vi "SIMCOMCommunicationTool_CF_vb.vi"(0 "VISA资源名称":refnum<visa-resource-name>="COM26", 1 "MSComm":refnum<k7>, 2 "MEID":string, 5 "通信协议名称":string, 9 "DelayTime":u32=100, 11 "error in":errorcluster, 12 "Debug":bool=TRUE, 14 "Slot":T1) -> (3 "CMD":string="发送 重启:AT+CRESET\r反馈:\r\nOK\r\n\r\n", 4 "字符串数值":bool=TRUE, 6 "反馈结果":bool=TRUE, 10 "ReturnData":string, 15 "error out":errorcluster)   [LabVIEW 2013]
doc: "本范例根据用户指示，对串口执行读写操作。范例运行时可按下“写入”或“读取”按钮，以及修改“读数”。\n\n设置的串口参数必须匹配连接仪器或设备的参数。本范例中，“读数”参数可指定串口读取的字节数。如端口字节超过指定的字节数，超出部分将不会被读取。如端口字节数少于指定的字节数，将返回超时错误。\n\n本范例可扩展流控制选项以包括XON和XOFF，从而允许用户选择控制字符。同时，用户可启用或禁用中止符。部分设备需要通过终止符确定命令字符串的结束位置。部分设备将发送终止符以说明待读取数据的末端。本范例演示了缓冲区中检测到终止符时，结束“读取”操作或添加终止符至“写入”数据末端的方法。"
uses:
  SystemCode/SysControl/Slot.ctl
  <vilib>/Utility/NIReport.llb/NI_report.lvclass
  SourceCode/GlobalValue.vi
  <vilib>/Utility/error.llb/Error Cluster From Error Code.vi
  <vilib>/addons/_office/excel.llb/Excel Get Data ([str]).vi
  <vilib>/ErrorRing/Error Ring.xnode
  <vilib>/addons/_office/NI_ReportGenerationToolkit.lvlib
  <vilib>/Utility/NIReport.llb/Excel/NI_Excel.lvclass
panel:
  out "Data":string[][](array[string])=[["8986031490021881534", "460036161669975", "2A645416CB435F94", "8006A127", "460036161669975@mycdma.cn", "DB60264368A1D188", "18101891253", "A1000021A59070"], ["8986031490021881535", "460036161669976", "32FA5764D69C76BE", "80FAE4E6", "460036161669976@mycdma.cn", "B3AA1B3D2F0D5593", "18964872399", "A1000021A58D61"], ["", "", "", "", "", "", "", ""], ["", "", "", "", "", "", "", ""], ["", "", "", "", "", "", "", ""], ["", "", "", "", "", "", "", ""], ["", "", "", "", "", "", "", ""], ["", "", "", "", "", "", "", ""], ["", "", "", "", "", "", "", ""], ["", "", "", "", "", "", "", ""], ["", "各位，模块烧号主要是写五码，包括IMSI、AKEY、MEID（ESN）、AN(EVDO USER)、AAA(EVDO PWD)。", "", "", "", "", "", ""], ["", "其中ESN和MEID在模块出厂时已经写入，两者均可通过AT指令读取，但ESN不可更改。", "", "", "", "", "", ""], ["", "经询问及实际测试，上海电信绑定ESN号而广东电信未绑定，意味着上海电信五码烧录到其它模块是不可用的，但广东电信则无此限制。", "", "", "", "", "", ""], ["", "", "", "", "", "", "", ""], ["", "", "", "", "", "", "", ""], ["", "目前已确定跟上海电信合作，后续模块及卡号使用过程中，如遇到模块损坏，则意味着该卡必须销号（除非向电信申请绑定新的ESN），否则烧录到其它模块中是没用的。", "", "", "", "", "", ""]]
  in  "命令列表":u16(ring)=18 items=["查询RTRECF", "设置RTRECF", "查询MEID", "设置MEID", "查询ESN", "设置ESN", "查询AKEY", "设置AKEY", "查询IMSI1", "设置IMSI1", "查询IMSI2", "设置IMSI2", "查询IMSI3", "设置IMSI3", "设置EVDO账号", "设置EVDO密码", "打开音频LOOPBACK", "关闭音频LOOPBACK", "重启", "打开网络", "查询网络状态", "连网测试", "查询CIP", "切换声音通道", "测试登录", "拨号", "挂断", "查询IP", "AT+CSOCKAUTHNV", "AT+CSOCKAUTH", "查询2G信号", "查询3G信号", "H330测试通讯", "H330打开音频回环", "H330关闭音频回环", "H330拨号"]
  out "ConfigPath":string="D:\\导航\\T-BOX\\新建文件夹\\config\\通信协议.xls"
  out "DataType":string="AT+CRESET"
  out "命令":string="AT+CRESET\r"
  out "响应":string="\r\nOK\r\n"
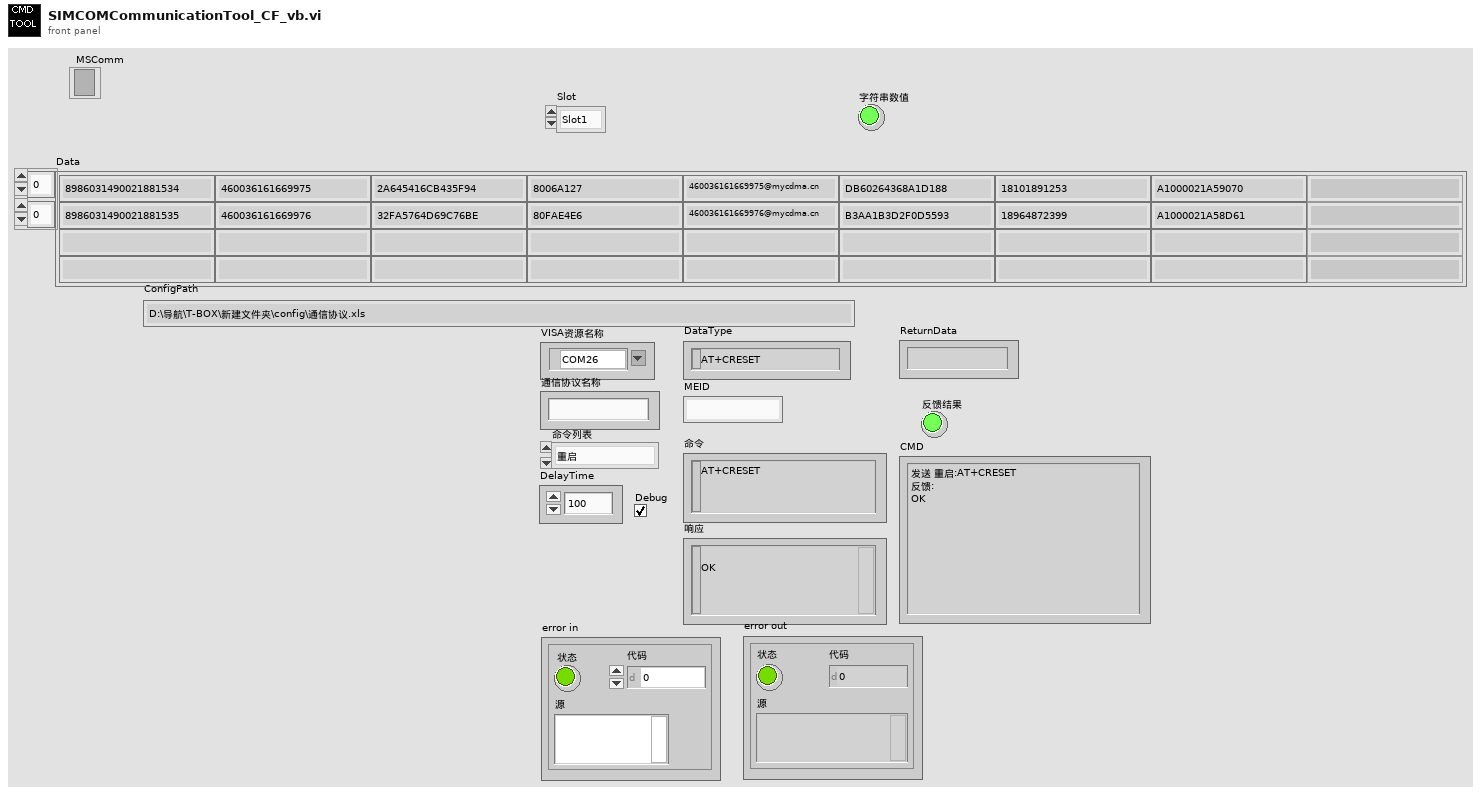
[diagram p1: front panel]
types:
  T1 = typedef "Slot.ctl" = enum16{"Slot1", "Slot2", "Slot3", "Slot4"}
  T2 = enum32{"invalid app kind", "Development System", "Run Time System", "Student Edition", "Embedded LabVIEW", "Evaluation", "Custom"}
  T3 = enum16{"maximized", "minimized", "normal", "no change"}
  T4 = enum16{"Standard Report", "HTML", "Word", "Excel"}
  T5 = cluster{"IMSI":string, "AKEY":string, "ESN":string, "EVDO账号":string, "EVDO密码":string, "设备号":string}
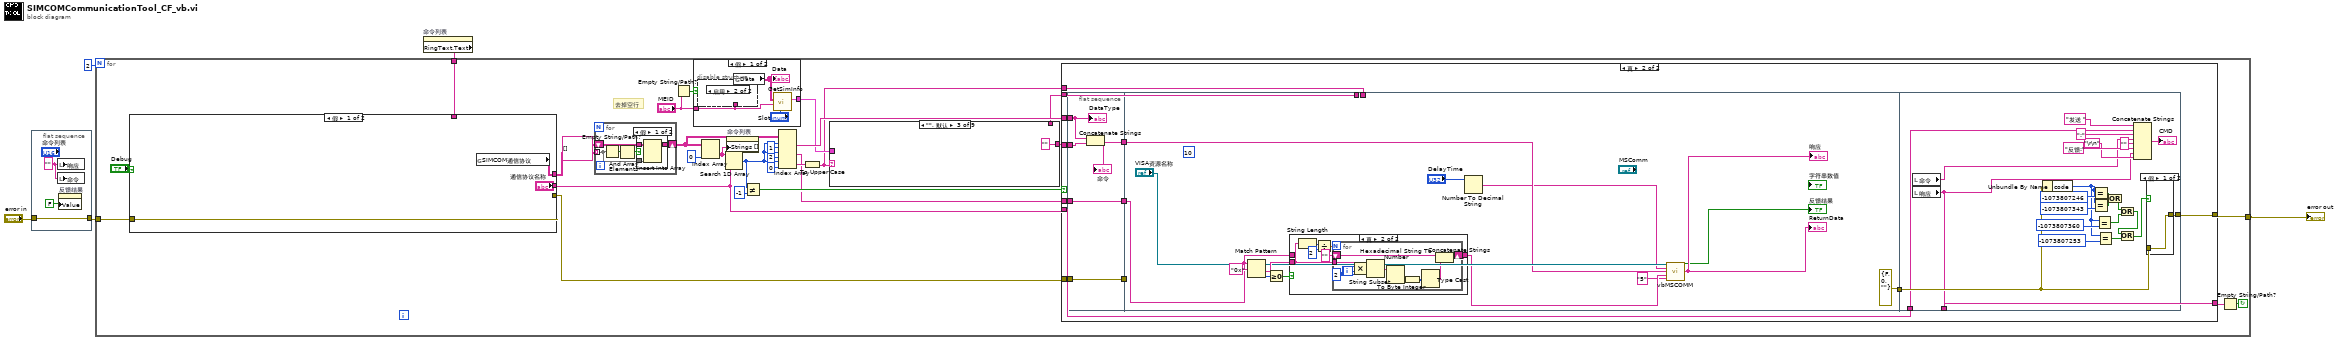
[diagram p0: block diagram]
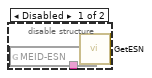
[diagram p2: hidden frame]
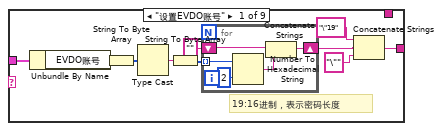
[diagram p5: hidden frame]
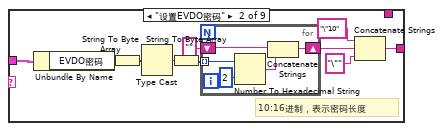
[diagram p6: hidden frame]
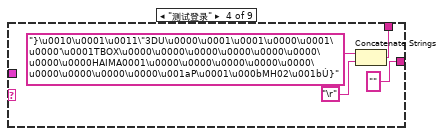
[diagram p7: hidden frame]
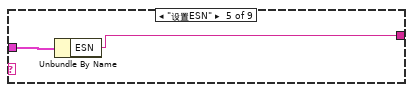
[diagram p8: hidden frame]
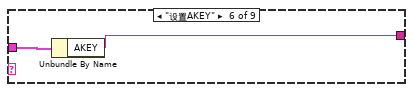
[diagram p9: hidden frame]
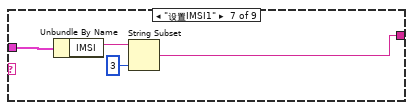
[diagram p10: hidden frame]
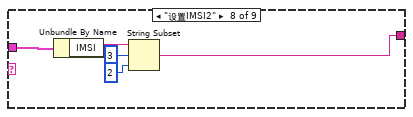
[diagram p11: hidden frame]
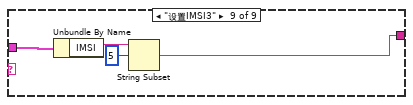
[diagram p12: hidden frame]
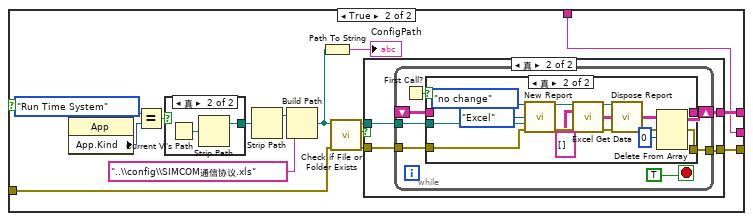
[diagram p13: hidden frame]
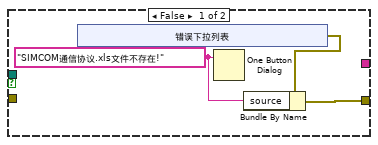
[diagram p14: hidden frame]
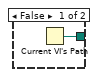
[diagram p16: hidden frame]
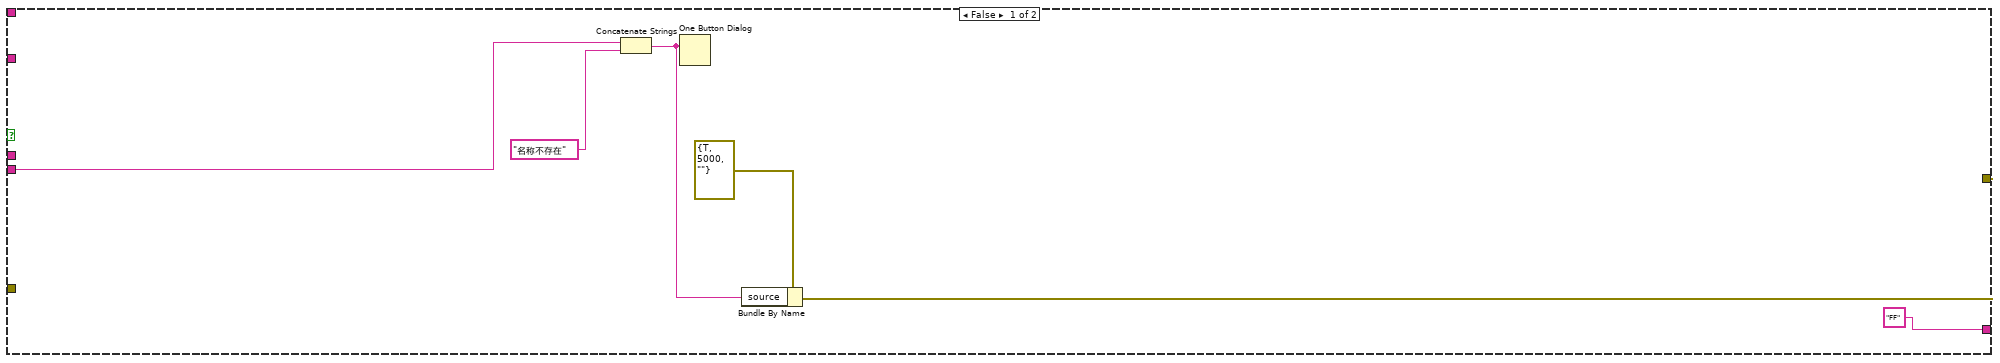
[diagram p17: hidden frame]
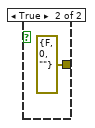
[diagram p19: hidden frame]
diagram:
  n1 = flat-sequence {
    tunnel: "error in" -> [w7]
    tunnel: [w7] -> w2
    frame #0 {
      w8 = "" ("响应")
      n2 = local write "响应"(w8) -> ()
      n3 = local write "命令"(w8) -> ()
      n4 = property on="反馈结果" class="Bool (严格)"("Value"=FALSE ("反馈结果")) -> ()  [unwired: 2 in, 2 out]
    }
  }
  n5 = property on="命令列表" class="Ring (严格)"() -> ("RingText.Text"=w1:string)  [unwired: 2 in, 2 out]
  n6 = for {
    N: 2 -> [_]
    tunnel: w2 -> [w24]
    tunnel: [w36] -> w5
    tunnel: w1 -> [w17]
    stop <- w22 continue-if-true
    # "去掉空行"
    n7 = case shown="假" "Debug" {
      tunnel: [w105 w110] -> w35
      tunnel: w24 -> [w105 w109]
      tunnel: ["通信协议名称" w107] -> w28
      tunnel: [w104 w108] -> w19
      tunnel: w17 -> [_ w107]
      frame False {
        n8 = global read "GlobalValue.vi" "SIMCOM通信协议"() -> (w104:string[][])
      }
      frame True {
        n9 = property class="App"() -> ("App.Kind"=w119:T2)  [unwired: 2 in, 2 out]
        n10 = Equal?(x=T2."Run Time System" ("y"), y=w119) -> (x = y?=w121:bool)
        n11 = case shown="真" w121 {
          tunnel: [w155 w157] -> w120
          frame False {
            n12 = Current VI's Path() -> (path=w155:path)
          }
          frame True {
            n13 = Current VI's Path() -> (path=w156:path)
            n14 = Strip Path(path=w156) -> (stripped path=w157:path)  [unwired: 1 out]
          }
        }
        n15 = Strip Path(path=w120) -> (stripped path=w114:path)  [unwired: 1 out]
        n16 = Build Path(base path=w114, name or relative path="..\\config\\SIMCOM通信协议.xls" ("连接的字符串")) -> (appended path=w116:path)
        n17 = Path To String(path=w116) -> (string=→"ConfigPath":string)
        n18 = call <vilib>:"Check if File or Folder Exists.vi"("error in (no error)"=w109, "path"=w116) -> ("error out"=w111:errorcluster, "file or folder exists?"=w113:bool, "dup path"=w112:path)  [unwired: 7 out]
        n19 = case shown="真" w113 {
          tunnel: w112 -> [_ w132]
          tunnel: w111 -> [_ w131]
          tunnel: [w123 w130] -> w110
          tunnel: [_ w129] -> w108
          frame False {
            w124 = "SIMCOM通信协议.xls文件不存在!" ("消息")
            n20 = xnode "错误下拉列表"() -> ("错误输出"=w122:errorcluster)
            n21 = One Button Dialog(message=w124) -> ()  [unwired: 1 in, 1 out]
            n22 = Bundle By Name(cluster=w122, "source"=w124) -> (w123:errorcluster)
          }
          frame True {
            n23 = while {
              tunnel: w132 -> [w138]
              tunnel: [w137] -> w130
              tunnel: w131 -> [w136]
              shift-right: [w139] -> w129
              shift-left: _ -> [w134]
              stop <- TRUE stop-if-true
              n24 = First Call?() -> (First Call?: T/F=w133:bool)
              n25 = case shown="真" w133 {
                tunnel: [w141 w145] -> w139
                tunnel: w138 -> [_ w144]
                tunnel: [w140 w143] -> w137
                tunnel: w136 -> [w140 w142]
                tunnel: w134 -> [w141 _]
                frame False {
                }
                frame True {
                  n26 = call <vilib>:"New Report.vi"("window state (normal)"=T3."no change", "report type"=T4."Excel", "template (empty)"=w144, "error in (no error)"=w142) -> ("report out"=w150:refnum<class "NI_report.lvclass">, "error out"=w151:errorcluster)  [unwired: 2 in, 8 out]
                  n27 = call-poly <vilib>:"Excel Get Data.vi"("report in"=w150, "data type"=string[][] [], "error in (no error)"=w151) -> ("report out"=w147:refnum<class "NI_report.lvclass">, "data"=w152:string[][], "error out"=w146:errorcluster)  [unwired: 10 in]
                  n28 = call-dynamic "Dispose Report.vi"("report in"=w147, "error in (no error)"=w146) -> ("error out"=w143:errorcluster)  [unwired: 3 in, 10 out]
                  n29 = Delete From Array(array=w152, index (row)=0 ("索引 (行)")) -> (array with subset deleted=w145:string[][])  [unwired: 2 in, 1 out]
                }
              }
            }
          }
        }
      }
    }
    n30 = for {
      tunnel: w19 -> [w43] mode=indexing
      shift-right: [w46] -> w18
      shift-left: string[][] [] -> [w47]
      n31 = Empty String/Path?(string/path=w43) -> (empty?=w45:bool[])
      n32 = And Array Elements(Boolean array=w45) -> (logical AND=w44:bool)
      n33 = case shown="假" w44 {
        tunnel: w47 -> [w50 w51]
        tunnel: [w49 w51] -> w46
        tunnel: w43 -> [w48 _]
        frame False {
          n34 = Insert Into Array(array=w50, new element=w48) -> (w49:string[][])  [unwired: 2 in]
        }
        frame True {
        }
      }
    }
    n35 = Empty String/Path?(string/path="MEID") -> (empty?=w10:bool)
    n36 = case shown="假" w10 {
      tunnel: [w40 _] -> w14
      tunnel: "MEID" -> [w37 _]
      frame False {
        n37 = disable-structure shown="启用" {
          disable-tunnel: w37 -> [w41 _]
          frame Disabled {
            n38 = global read "GlobalValue.vi" "MEID-ESN"() -> (w42:string[][])
            n39 = call "GetESN.vi"("MEID"=w41, "Data"=w42) -> ()  [unwired: 9 in, 1 out]
          }
          frame Enabled {
          }
        }
        n40 = global read "GlobalValue.vi" "Data"() -> (w39:string[][])
        "Data" <- w39
        n41 = call "GetSimInfo.vi"("Slot"="Slot", "MEID"=w37, "Data"=w39) -> ("SIMInfo"=w40:T5)  [unwired: 6 in, 2 out]
      }
      frame True {
      }
    }
    n42 = Index Array(array=w18, index (col)=0 ("禁用的索引 (列)")) -> (element=w26:string[])  [unwired: 1 in]
    n43 = Search 1D Array(1D array=w26, element=w28) -> (index of element=w21:i32)  [unwired: 1 in]
    n44 = property on="命令列表" class="Ring (严格)"("Strings []"=w26) -> ()  [unwired: 2 in, 2 out]
    n45 = Not Equal?(x=w21, y=-1) -> (x != y?=w30:bool)
    n46 = Index Array(array=w18, index (row) #1=w21, index (col) #1=1 ("索引 (列)"), index (row) #2=w21, index (col) #2=2 ("索引 (列)"), index (row) #3=w21, index (col) #3=0 ("索引 (列)")) -> (element #1=w15:string, element #2=w11:string, element #3=w16:string)
    n47 = To Upper Case(1:w16) -> (0:w12:string)
    n48 = case shown="\"\", 默认" w12 {
      tunnel: [w54 w69 "" "" ("IMSI") w87 w89 w91 w96 w101] -> w29
      tunnel: w14 -> [w53 w67 _ _ w88 w90 w94 w99 w103]
      tunnel: [_ _ _ w83 _ _ _ _ _] -> w13
      frame "设置EVDO账号" {
        # "19:16进制，表示密码长度"
        n49 = Unbundle By Name(w53) -> ("EVDO账号"=w52:string)
        n50 = String To Byte Array(string=w52) -> (unsigned byte array=w61:u8[])
        n51 = Type Cast(x=w61) -> (*(type *) &x=w59:string)  [unwired: 1 in]
        n52 = String To Byte Array(string=w59) -> (unsigned byte array=w60:u8[])
        n53 = for {
          tunnel: w60 -> [w66] mode=indexing
          shift-right: [w64] -> w55
          shift-left: "" -> [w63]
          n54 = Number To Hexadecimal String(1:i16 2 ("宽度(-)"), 2:w66) -> (0:w65:string)
          n55 = Concatenate Strings(w63, w65) -> (w64:string)
        }
        n56 = Concatenate Strings("\"19" ("字符串"), w55, "\"" ("字符串")) -> (w54:string)
      }
      frame "设置EVDO密码" {
        # "10:16进制，表示密码长度"
        n57 = Unbundle By Name(w67) -> ("EVDO密码"=w68:string)
        n58 = String To Byte Array(string=w68) -> (unsigned byte array=w76:u8[])
        n59 = Type Cast(x=w76) -> (*(type *) &x=w74:string)  [unwired: 1 in]
        n60 = String To Byte Array(string=w74) -> (unsigned byte array=w75:u8[])
        n61 = for {
          tunnel: w75 -> [w81] mode=indexing
          shift-right: [w79] -> w72
          shift-left: "" -> [w78]
          n62 = Number To Hexadecimal String(1:i16 2 ("宽度(-)"), 2:w81) -> (0:w80:string)
          n63 = Concatenate Strings(w78, w80) -> (w79:string)
        }
        n64 = Concatenate Strings("\"10" ("字符串"), w72, "\"" ("字符串")) -> (w69:string)
      }
      frame "", Default {
      }
      frame "测试登录" {
        n65 = Concatenate Strings("}\u0010\u0001\u0011\"3DU\u0000\u0001\u0001\u0000\u0001\u0000'\u0001TBOX\u0000\u0000\u0000\u0000\u0000\u0000\u0000\u0000HAIMA0001\u0000\u0000\u0000\u0000\u0000\u0000\u0000\u0000\u0000\u001aP\u0001\u000bMH02\u001bÚ}" ("字符串"), "\r") -> (w83:string)
      }
      frame "设置ESN" {
        n66 = Unbundle By Name(w88) -> ("ESN"=w87:string)
      }
      frame "设置AKEY" {
        n67 = Unbundle By Name(w90) -> ("AKEY"=w89:string)
      }
      frame "设置IMSI1" {
        n68 = Unbundle By Name(w94) -> ("IMSI"=w93:string)
        n69 = String Subset(string=w93, length (rest)=3 ("长度（剩余）")) -> (substring=w91:string)  [unwired: 1 in]
      }
      frame "设置IMSI2" {
        n70 = Unbundle By Name(w99) -> ("IMSI"=w98:string)
        n71 = String Subset(string=w98, offset (0)=3 ("偏移量(0)"), length (rest)=2 ("长度（剩余）")) -> (substring=w96:string)
      }
      frame "设置IMSI3" {
        n72 = Unbundle By Name(w103) -> ("IMSI"=w102:string)
        n73 = String Subset(string=w102, offset (0)=5 ("偏移量(0)")) -> (substring=w101:string)  [unwired: 1 in]
      }
    }
    n74 = case shown="真" w30 {
      tunnel: w28 -> [w163 w169]
      tunnel: w15 -> [_ w176]
      tunnel: w29 -> [_ w175]
      tunnel: w35 -> [_ w174]
      tunnel: [w159 w172] -> w36
      tunnel: ["FF" ("响应") w171] -> w23
      tunnel: w13 -> [_ w168]
      tunnel: w12 -> [_ w167]
      tunnel: w11 -> [_ w166]
      frame False {
        n75 = Concatenate Strings(w163, "名称不存在" ("消息")) -> (w160:string)
        n76 = One Button Dialog(message=w160) -> ()  [unwired: 1 in, 1 out]
        n77 = Bundle By Name(cluster=errorcluster {"status"=TRUE, "code"=5000, "source"=""} ("error in 1 (no error)"), "source"=w160) -> (w159:errorcluster)
      }
      frame True {
        n78 = flat-sequence {
          tunnel: w176 -> [w180]
          tunnel: w175 -> [w179]
          tunnel: w174 -> [w181]
          tunnel: [w181] -> w173
          tunnel: [w178] -> w170
          tunnel: w166 -> [w177]
          tunnel: [w177] -> w165
          tunnel: w173 -> [_]
          tunnel: w170 -> [w189]
          tunnel: w168 -> [_]
          tunnel: w167 -> [_]
          tunnel: w165 -> [w191]
          tunnel: [errorcluster {"status"=FALSE, "code"=0, "source"=""} ("错误输出")] -> w164
          tunnel: [w229] -> w172
          tunnel: w169 -> [w225]
          tunnel: [w219] -> w171
          tunnel: w164 -> [w228]
          frame #0 {
            n79 = Concatenate Strings(w180, w179) -> (w178:string)
            "命令" <- w178
            "DataType" <- w180
          }
          frame #1 {
            (unwired) 10
            n80 = Match Pattern(string=w191, regular expression="0x" ("正则表达式")) -> (after substring=w193:string, offset past match=w194:i32)  [unwired: 1 in, 2 out]
            n81 = Greater Or Equal To 0?(x=w194) -> (x >= 0?=w192:bool)
            n82 = case shown="真" w192 {
              tunnel: w193 -> [_ w198]
              tunnel: [w196 w197] -> w186
              tunnel: w191 -> [w196 _]
              frame False {
              }
              frame True {
                n83 = String Length(string=w198) -> (length=w201:i32)
                n84 = Divide(x=w201, y=2) -> (x/y=w199:dbl)
                n85 = for {
                  N: w199 -> [_]
                  tunnel: w198 -> [w207]
                  shift-right: [w209] -> w197
                  shift-left: "" -> [w208]
                  i -> [w205]
                  w203 = 2 ("x")
                  n86 = Multiply(x=w203, y=w205) -> (x*y=w204:i32)
                  n87 = String Subset(string=w207, offset (0)=w204, length (rest)=w203) -> (substring=w206:string)
                  n88 = Hexadecimal String To Number(string=w206) -> (number=w212:u32)  [unwired: 2 in, 1 out]
                  n89 = To Byte Integer(number=w212) -> (8bit integer=w211:i8)
                  n90 = Type Cast(x=w211) -> (*(type *) &x=w210:string)  [unwired: 1 in]
                  n91 = Concatenate Strings(w208, w210) -> (w209:string)
                }
              }
            }
            n92 = Number To Decimal String(number="DelayTime") -> (decimal integer string=w187:string)  [unwired: 1 in]
            n93 = call "vbMSCOMM.vi"("端口号"="VISA资源名称", "Send Delay(ms)"=w187, "Send Data"=w189, "Data Return"=w186, "cycle times"="5") -> ("result"=→"反馈结果":bool, "Rec Data"=→"ReturnData" →"响应":string)  [unwired: 9 in]
          }
          frame #2 {
            n94 = local read "命令"() -> (w220:string)
            n95 = local read "响应"() -> (w219:string)
            n96 = Unbundle By Name(w228) -> ("code"=w217:i32)
            n97 = Equal?(x=w217, y=-1073807246) -> (x = y?=w226:bool)
            n98 = Equal?(x=w217, y=-1073807343) -> (x = y?=w223:bool)
            n99 = Equal?(x=w217, y=-1073807360) -> (x = y?=w221:bool)
            n100 = Equal?(x=w217, y=-1073807253) -> (x = y?=w214:bool)
            n101 = Or(x=w226, y=w223) -> (x .or. y?=w222:bool)
            n102 = Or(x=w222, y=w221) -> (x .or. y?=w215:bool)
            n103 = Or(x=w215, y=w214) -> (x .or. y?=w213:bool)
            n104 = Concatenate Strings("发送 " ("字符串"), w225, ":" ("字符串"), w220, "" ("字符串"), "反馈:" ("字符串"), w219, "\r\n") -> (→"CMD":string)
            n105 = case shown="假" w213 {
              tunnel: [w236 errorcluster {"status"=FALSE, "code"=0, "source"=""} ("t")] -> w229
              tunnel: w228 -> [w236 _]
              frame False {
              }
              frame True {
              }
            }
          }
        }
      }
    }
    n106 = Empty String/Path?(string/path=w23) -> (empty?=w22:bool)
  }
  "error out" <- w5
